vi "Read Startup INI.vi"(8 "error in (no error)":errorcluster, 11 "Startup INI file":path=path "C:/Projects/Ichor/AVC2/startup.ini") -> (0 "error out":errorcluster, 2 "Startup INI":T1={"ConfigFolder"=path "C:/AVC2/Config", "DataLogFolder"=path "C:/AVC2/DataLog", "SystemLogFolder"=path "C:/AVC2/SystemLog", "SequenceFolder"=path "C:/AVC2/SeqFolder", "MainStartup"="MainProcess.vi", "MainUI"="AVC2_Eng_MainUI.vi", "AppConfigFilename"="AVC2_Config.ini", "IOConfigFilename"="IOConfig.xml", "SystemSimulation"=FALSE, "DLPUIConfigFilename"="", "DLP2InitializationFilePath"=path "", "RecipeXMLFolder"=path "", "CalibrationRecipeXMLFolder"=path ""}, 4 "default file created":bool)   [LabVIEW 2022 SP3]
doc: "Developed by Kevin Thompson\nkevin@thompsonengineering.net\n\nCopyright 2018-2020\nThompson Engineering, LLC"
uses:
  DataTypes/Startup INI Data--cluster.ctl
  <userlib>/_OpenG.lib/file/file.llb/File Exists - Scalar__ogtk.vi
  <vilib>/Utility/config.llb/NI_LVConfig.lvlib
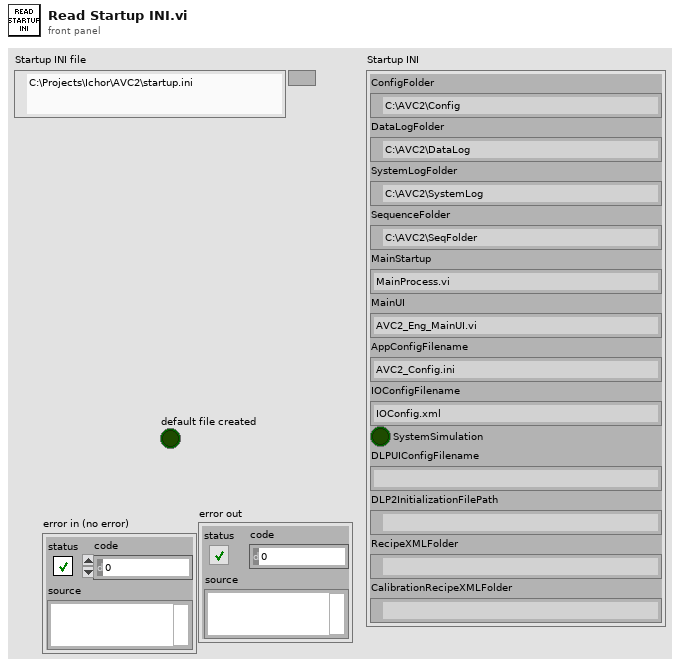
[diagram p1: front panel]
types:
  T1 = typedef "Startup INI Data--cluster.ctl" = cluster{"ConfigFolder":path, "DataLogFolder":path, "SystemLogFolder":path, "SequenceFolder":path, "MainStartup":string, "MainUI":string, "AppConfigFilename":string, "IOConfigFilename":string, "SystemSimulation":bool, "DLPUIConfigFilename":string, "DLP2InitializationFilePath":path, "RecipeXMLFolder":path, "CalibrationRecipeXMLFolder":path}
  T2 = typedef "NI_LVConfig.lvlib/Config Data RefNum.ctl" = refnum<k1>
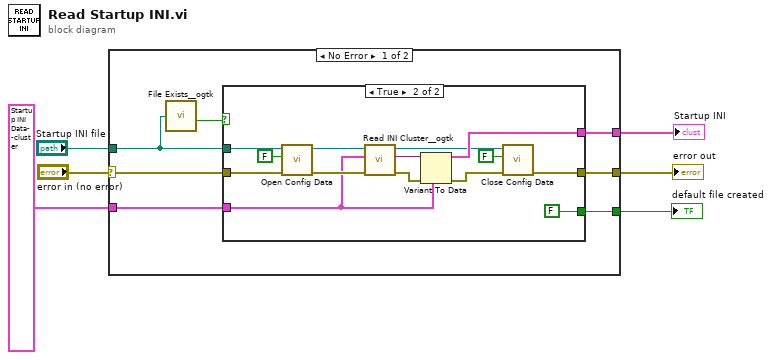
[diagram p0: block diagram]
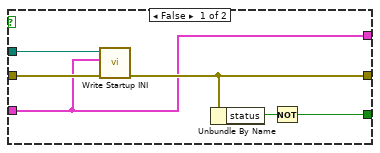
[diagram p2: hidden frame]
diagram:
  n1 = case shown="No Error" "error in (no error)" {
    selector: "error in (no error)" -> [w8 w34]
    tunnel: [w12 _] -> w6
    tunnel: [w11 w34] -> w5
    tunnel: [w10 _] -> w4
    tunnel: "Startup INI file" -> [w9 _]
    tunnel: T1 {"ConfigFolder"=path "C:/AVC2/Config", "DataLogFolder"=path "C:/AVC2/DataLog", "SystemLogFolder"=path "C:/AVC2/SystemLog", "SequenceFolder"=path "C:/AVC2/SeqFolder", "MainStartup"="MainProcess.vi", "MainUI"="AVC2_MainUI.vi", "AppConfigFilename"="AVC2_Config.ini", "IOConfigFilename"="IOConfig.xml", "SystemSimulation"=FALSE, "DLPUIConfigFilename"="", "DLP2InitializationFilePath"=path "", "RecipeXMLFolder"=path "", "CalibrationRecipeXMLFolder"=path ""} ("Startup INI") -> [w7 _]
    frame No Error {
      n2 = call-poly <userlib>:"File Exists__ogtk.vi"("file path"=w9) -> ("exists"=w13:bool)  [unwired: 6 in, 1 out]
      n3 = case shown="True" w13 {
        tunnel: w9 -> [w17 w33]
        tunnel: [w14 w32] -> w12
        tunnel: [w15 w31] -> w11
        tunnel: w8 -> [w16 w24]
        tunnel: w7 -> [w14 w23]
        tunnel: [w18 FALSE] -> w10
        frame False {
          n4 = call "Write Startup INI.vi"("error in (no error)"=w16, "Startup INI"=w14, "Startup INI file"=w17) -> ("error out"=w15:errorcluster)  [unwired: 8 in]
          n5 = Unbundle By Name(w15) -> ("status"=w19:bool)
          n6 = Not(x=w19) -> (.not. x?=w18:bool)
        }
        frame True {
          n7 = call <vilib>:"Open Config Data.vi"("error in (no error)"=w24, "create file if necessary (T)"=FALSE, "configuration file path"=w33) -> ("error out"=w29:errorcluster, "refnum"=w30:T2)  [unwired: 6 in, 1 out]
          n8 = call <userlib>:"Read INI Cluster__ogtk.vi"("error in (no error)"=w29, "INI Fomatted Cluster Type"=w23, "refnum"=w30) -> ("error out"=w27:errorcluster, "INI Fomatted Cluster"=w25:variant, "dup refnum"=w28:T2)  [unwired: 4 in, 2 out]
          n9 = Variant To Data(error in=w27, type=w23, Variant=w25) -> (data=w32:T1, error out=w26:errorcluster)
          n10 = call <vilib>:"Close Config Data.vi"("error in (no error)"=w26, "write file if changed (T)"=FALSE, "refnum"=w28) -> ("error out"=w31:errorcluster)  [unwired: 7 in, 1 out]
        }
      }
    }
    frame Error {
    }
  }
  "Startup INI" <- w6
  "error out" <- w5
  "default file created" <- w4
